vi "Write Key (Variant)__lvcfg.vi"(5 "float number format":string, 6 "write raw string? (F)":bool, 7 "section":string, 8 "error in (no error)":errorcluster, 9 "key-value":variant, 10 "key (optional)":string, 11 "Config in":T1) -> (0 "error out":errorcluster, 3 "Config out":T1)   [LabVIEW 2017, in "LabVIEW Config(Variant).lvlib"]
doc: "Writes a value associated with key in a specified section of the configuration data identified by refnum. If \"key\" input is not specified, the name of the variant object is used as the key.\n\nFor example a Boolean named \"Enable\" with a value of TRUE would correspond to the key-value pair:\n\nEnable=TRUE\n\nNote: Special characters in section and key names will be escape-coded. These include the following: \\00-\\1F (non-printable chars); \"[\", \"]\", and \"=\" (INI syntax elements); \\FE (\"þ\") and \\FF (\"ÿ\") (legacy bracket encoding); Additionally, the escape character, \"\\\", will be escaped as \"\\\\\"."
uses:
  LabVIEW Config(Variant).lvlib
  <userlib>/_NEVSTOP/Communicable State Machine(CSM)/addons/INI-Static-Variable-Support/LabVIEW-Config/Config.ctl
  <userlib>/_NEVSTOP/Communicable State Machine(CSM)/addons/INI-Static-Variable-Support/LabVIEW-Config/Write Key (Raw).vi
  <userlib>/_NEVSTOP/Communicable State Machine(CSM)/addons/INI-Static-Variable-Support/LabVIEW-Config/Write Key (String).vi
  <userlib>/_NEVSTOP/Communicable State Machine(CSM)/addons/INI-Static-Variable-Support/LabVIEW-Config/LabVIEW-Config.lvlib
  <userlib>/_NEVSTOP/Communicable State Machine(CSM)/Communicable State Machine.lvlib
panel:
  in  "Ref for recursive call":refnum<vi>
  # "Write Key (Variant).vi\n\nWrites a variant key-value to INI file.\n\nPlease visit http://www.OpenG.org to learn about the\nOpen Source LabVIEW software movement.\n\nNOTICE -- YOU MUST LEAVE THIS NOTICE IN PLACE.  PER THE TERMS OF THE LICENSE BELOW, YOU MAY SUBLICENSE THIS SOFTWARE \nIN ANY WAY THAT DOES NOT CONFLICT WITH THIS LICENSE.\n\n### BSD License (http://www.opensource.org/licenses/bsd-license.php) Begin ###\n \nCopyright (c) 2002, Jean-Pierre Drolet <drolet_jp@hotmail.com>\nCopyright (c) 2002-2006, Jim Kring <jim@jimkring.com>\n\nAll rights reserved.\n\nRedistribution and use in source and binary forms, with or without modification, are permitted provided that the following conditions are met:\n\n    * Redistributions of source code must retain the above copyright notice, this list of conditions and the following disclaimer.\n    * Redistributions in binary form must reproduce the above copyright notice, this list of conditions and the following disclaimer in the \n       documentation and/or other materials provided with the distribution.\n    * Neither the name of SciWare, James Kring, Inc., nor the names of its contributors may be used to endorse or promote products derived \n       from this software without specific prior written permission.\n\nTHIS SOFTWARE IS PROVIDED BY THE COPYRIGHT HOLDERS AND CONTRIBUTORS \"AS IS\" AND ANY EXPRESS OR IMPLIED WARRANTIES, \nINCLUDING, BUT NOT LIMITED TO, THE IMPLIED WARRANTIES OF MERCHANTABILITY AND FITNESS FOR A PARTICULAR PURPOSE ARE \nDISCLAIMED. IN NO EVENT SHALL THE COPYRIGHT OWNER OR CONTRIBUTORS BE LIABLE FOR ANY DIRECT, INDIRECT, INCIDENTAL,\n SPECIAL, EXEMPLARY, OR CONSEQUENTIAL DAMAGES (INCLUDING, BUT NOT LIMITED TO, PROCUREMENT OF SUBSTITUTE GOODS OR \nSERVICES; LOSS OF USE, DATA, OR PROFITS; OR BUSINESS INTERRUPTION) HOWEVER CAUSED AND ON ANY THEORY OF LIABILITY, \nWHETHER IN CONTRACT, STRICT LIABILITY, OR TORT (INCLUDING NEGLIGENCE OR OTHERWISE) ARISING IN ANY WAY OUT OF THE USE \nOF THIS SOFTWARE, EVEN IF ADVISED OF THE POSSIBILITY OF SUCH DAMAGE.\n\n### BSD License End ###"
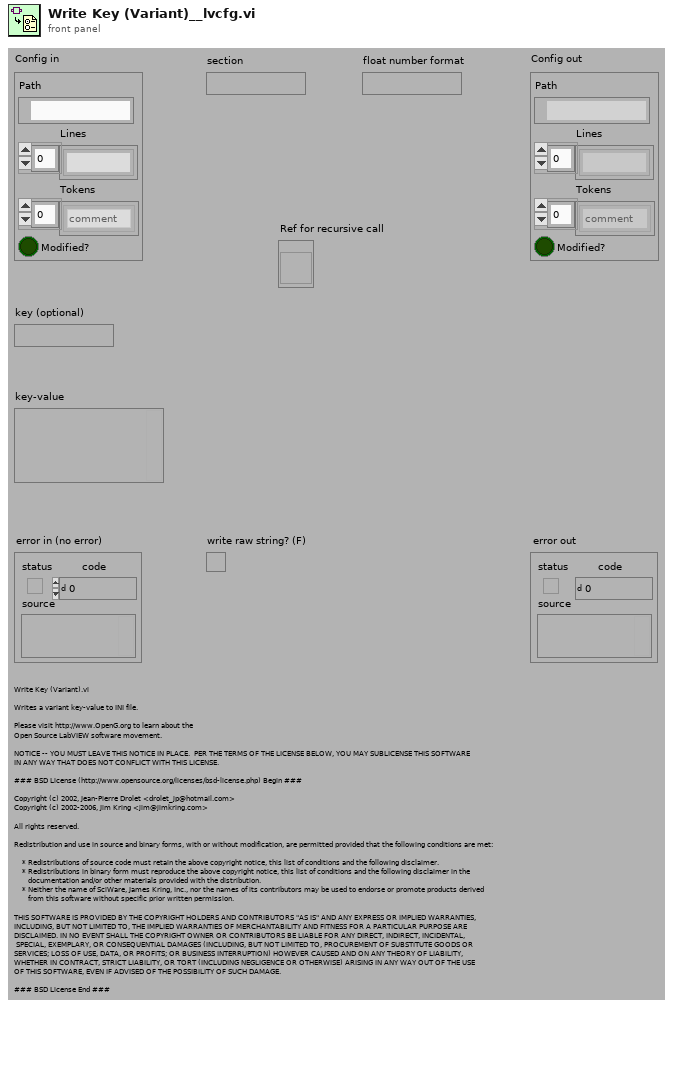
[diagram p1: front panel]
types:
  T1 = typedef "LabVIEW-Config.lvlib/Config.ctl" = cluster{"Path":path, "Lines":string[], "Tokens":enum8{"comment", "section", "key"}[], "Modified?":bool}
  T2 = typedef "Type Descriptor Enumeration__ogtk.ctl" = enum8{"<Null>", "I8", "I16", "I32", "I64", "U8", "U16", "U32", "U64", "SGL", "DBL", "EXT", "CSG", "CDB", "CXT", "0x0F", "0x10", "0x11", "0x12", "0x13", "0x14", "Enum U8", "Enum U16", "Enum U32", "Enum U64", "SGL PQ", "DBL PQ", "EXT PQ", "CSG PQ", "CDB PQ", "CXT PQ", "0x1F", "0x20", "Boolean", "0x22", "0x23", "0x24", "0x25", "0x26", "0x27", "0x28", "0x29", "0x2A", "0x2B", "0x2C", "0x2D", "0x2E", "0x2F", "String", "0x31", "Path", "Pict", "0x34", "0x35", "0x36", "DAQ", "0x38", "0x39", "0x3A", "0x3B", "0x3C", "0x3D", "0x3E", "0x3F", "Array", "0x41", "0x42", "0x43", "0x44", "0x45", "0x46", "0x47", "0x48", "0x49", "0x4A", "0x4B", "0x4C", "0x4D", "0x4E", "0x4F", "Cluster", "0x51", "0x52", "Variant", "Waveform", "0x55", "0x56", "0x57", "0x58", "0x59", "0x5A", "0x5B", "0x5C", "0x5D", "0x5E", "Fixed Point", "0x60", "0x61", "0x62", "0x63", "0x64", "0x65", "0x66", "0x67", "0x68", "0x69", "0x6A", "0x6B", "0x6C", "0x6D", "0x6E", "0x6F", "Refnum", "0x71", "0x72", "Set Collection", "Map Collection"}
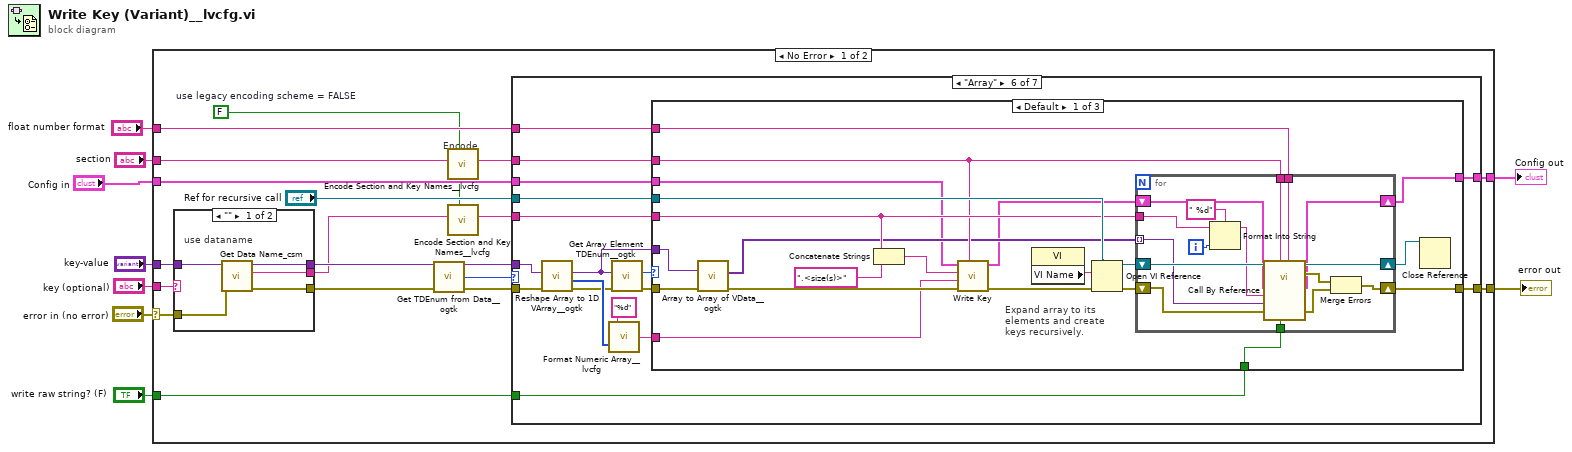
[diagram p0: block diagram]
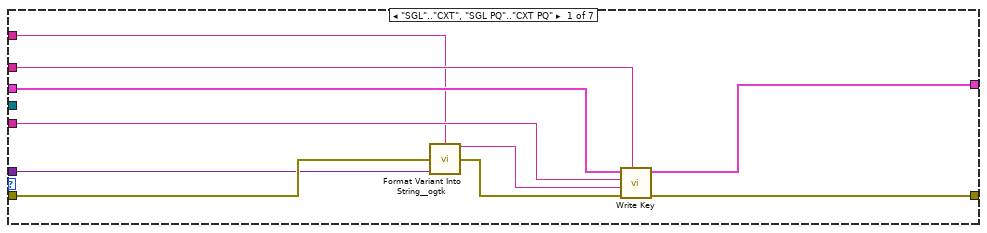
[diagram p2: hidden frame]
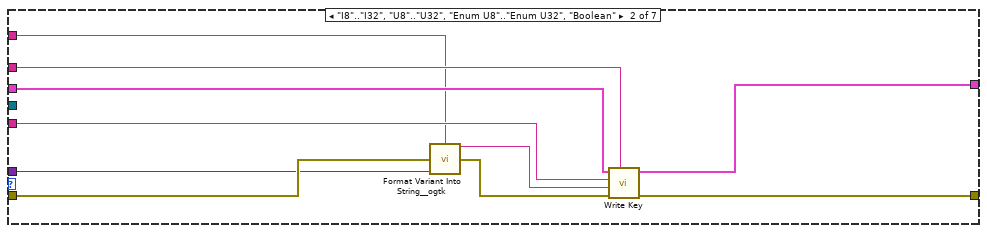
[diagram p3: hidden frame]
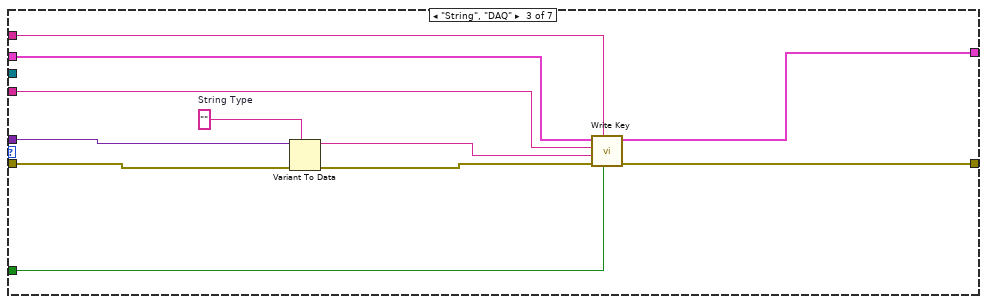
[diagram p4: hidden frame]
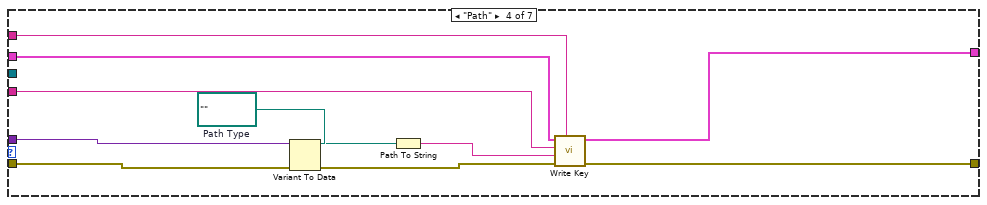
[diagram p5: hidden frame]
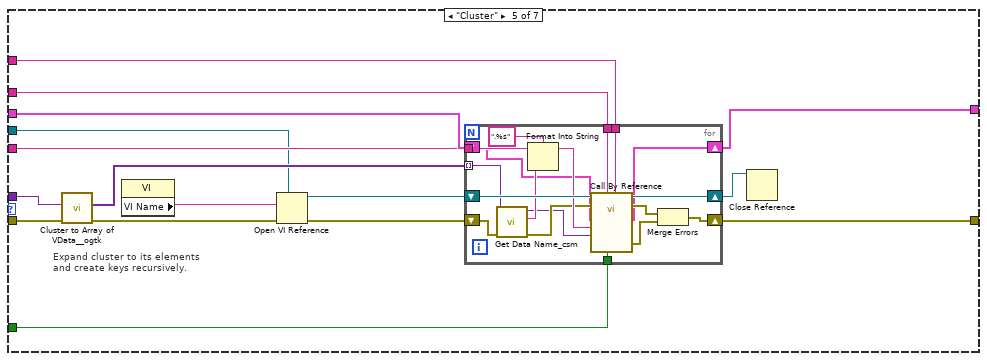
[diagram p6: hidden frame]
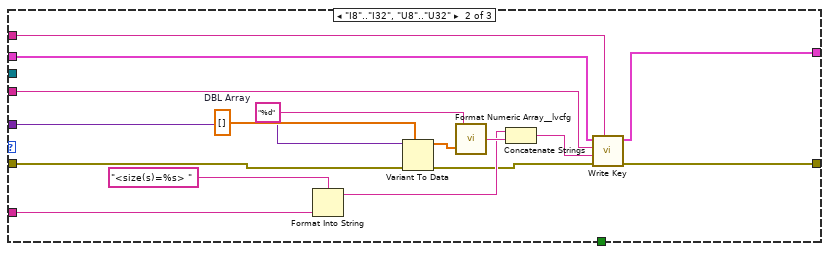
[diagram p7: hidden frame]
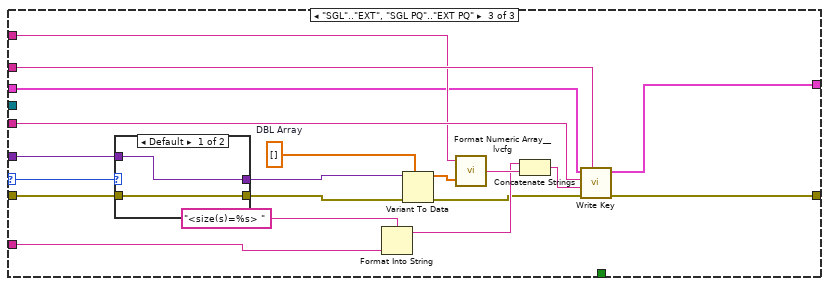
[diagram p8: hidden frame]
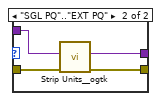
[diagram p9: hidden frame]
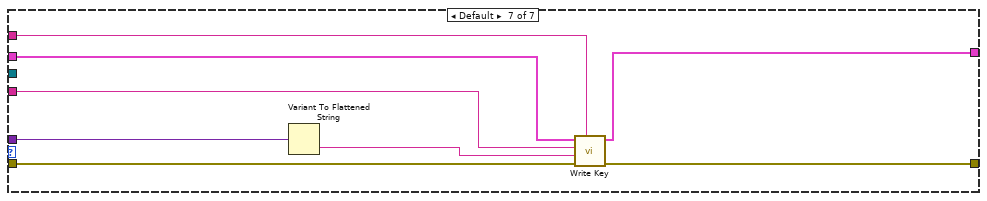
[diagram p10: hidden frame]
diagram:
  n1 = case shown="No Error" "error in (no error)" {
    selector: "error in (no error)" -> [w23 w215]
    tunnel: "Config in" -> [w26 w214]
    tunnel: [w25 w215] -> w9
    tunnel: "key-value" -> [w20 _]
    tunnel: "key (optional)" -> [w24 _]
    tunnel: "section" -> [w15 _]
    tunnel: "float number format" -> [w17 _]
    tunnel: "write raw string? (F)" -> [w16 _]
    tunnel: [w10 w214] -> w1
    frame No Error {
      w11 = FALSE  # use legacy encoding scheme = FALSE
      # "Encode"
      n2 = case shown="\"\"" w24 {
        selector: w24 -> [_ w213]
        tunnel: [w210 w213] -> w13
        tunnel: w20 -> [w207 w211]
        tunnel: w23 -> [w209 w212]
        tunnel: [w208 w212] -> w21
        tunnel: [w206 w211] -> w19
        frame "" {
          # "use dataname"
          n3 = call <userlib>:"Get Data Name_csm.vi"("error in (no error)"=w209, "Data"=w207) -> ("error out"=w208:errorcluster, "Data Name"=w210:string, "Data dup"=w206:variant)  [unwired: 7 in]
        }
        frame Default {
          # "use optional\nkey"
        }
      }
      n4 = call <userlib>:"Get TDEnum from Data__ogtk.vi"("Data"=w19) -> ("Type Descriptor Enumeration"=w22:T2)  [unwired: 4 in]
      n5 = call "Encode Section and Key Names__lvcfg.vi"("use legacy encoding scheme? (FALSE)"=w11, "string"=w15) -> ("encoded string"=w14:string)  [unwired: 9 in]
      n6 = call "Encode Section and Key Names__lvcfg.vi"("use legacy encoding scheme? (FALSE)"=w11, "string"=w13) -> ("encoded string"=w12:string)  [unwired: 9 in]
      n7 = case shown="\"Array\"" w22 {
        tunnel: w19 -> [w32 w42 w55 w67 w77 w117 w202]
        tunnel: w26 -> [w30 w39 w48 w60 w81 w111 w199]
        tunnel: [w36 w46 w53 w65 w79 w119 w205] -> w25
        tunnel: w21 -> [w33 w43 w52 w64 w76 w116 w201]
        tunnel: w12 -> [w35 w45 w51 w63 w73 w110 w204]
        tunnel: w14 -> [w34 w44 w50 w62 w80 w112 w203]
        tunnel: "Ref for recursive call" -> [_ _ _ _ w72 w118 _]
        tunnel: w17 -> [w27 w37 _ _ w71 w105 _]
        tunnel: w16 -> [_ _ w49 _ w70 w104 _]
        tunnel: [w28 w38 w47 w58 w69 w103 w198] -> w10
        frame "SGL".."CXT", "SGL PQ".."CXT PQ" {
          n8 = call <userlib>:"Format Variant Into String__ogtk.vi"("Format String"=w27, "error in (no error)"=w33, "Variant"=w32) -> ("Output String"=w29:string, "error out"=w31:errorcluster)  [unwired: 11 in]
          n9 = call-poly <userlib>:"Write Key.vi"("Section Name"=w34, "error in (no error)"=w31, "Value"=w29, "Key Name"=w35, "Config in"=w30) -> ("error out"=w36:errorcluster, "Config out"=w28:T1)  [unwired: 4 in, 1 out]
        }
        frame "I8".."I32", "U8".."U32", "Enum U8".."Enum U32", "Boolean" {
          n10 = call <userlib>:"Format Variant Into String__ogtk.vi"("Format String"=w37, "error in (no error)"=w43, "Variant"=w42) -> ("Output String"=w40:string, "error out"=w41:errorcluster)  [unwired: 11 in]
          n11 = call-poly <userlib>:"Write Key.vi"("Section Name"=w44, "error in (no error)"=w41, "Value"=w40, "Key Name"=w45, "Config in"=w39) -> ("error out"=w46:errorcluster, "Config out"=w38:T1)  [unwired: 4 in, 1 out]
        }
        frame "String", "DAQ" {
          w57 = ""  # String Type
          n12 = Variant To Data(error in=w52, type=w57, Variant=w55) -> (data=w56:string, error out=w54:errorcluster)
          n13 = call-poly <userlib>:"Write Key.vi"("Write Raw String? (F)"=w49, "Section Name"=w50, "error in (no error)"=w54, "Value"=w56, "Key Name"=w51, "Config in"=w48) -> ("error out"=w53:errorcluster, "Config out"=w47:T1)  [unwired: 3 in, 1 out]
        }
        frame "Path" {
          w68 = path ""  # Path Type
          n14 = Variant To Data(error in=w64, type=w68, Variant=w67) -> (data=w61:path, error out=w66:errorcluster)
          n15 = Path To String(path=w61) -> (string=w59:string)
          n16 = call-poly <userlib>:"Write Key.vi"("Section Name"=w62, "error in (no error)"=w66, "Value"=w59, "Key Name"=w63, "Config in"=w60) -> ("error out"=w65:errorcluster, "Config out"=w58:T1)  [unwired: 4 in, 1 out]
        }
        frame "Cluster" {
          # "Expand cluster to its elements\nand create keys recursively."
          n17 = call <userlib>:"Cluster to Array of VData__ogtk.vi"("error in (no error)"=w76, "Cluster"=w77) -> ("error out"=w74:errorcluster, "Array of VData"=w75:variant[])  [unwired: 8 in]
          n18 = property class="VI"() -> ("VI Name"=w78:string)  [unwired: 2 in, 2 out]
          n19 = Open VI Reference(type specifier VI Refnum (for type only)=w72, vi path=w78, error in (no error)=w74) -> (vi reference=w84:refnum<vi>, error out=w82:errorcluster)  [unwired: 3 in]
          n20 = for {
            shift-right: [w101] -> w83
            shift-left: w84 -> [w102]
            shift-right: [w97] -> w79
            shift-left: w82 -> [w92]
            tunnel: w75 -> [w90] mode=indexing
            tunnel: w80 -> [w100]
            tunnel: w73 -> [w96]
            tunnel: w71 -> [w88]
            tunnel: w70 -> [w86]
            shift-right: [w85] -> w69
            shift-left: w81 -> [w87]
            n21 = call <userlib>:"Get Data Name_csm.vi"("error in (no error)"=w92, "Data"=w90) -> ("error out"=w91:errorcluster, "Data Name"=w95:string, "Data dup"=w89:variant)  [unwired: 7 in]
            n22 = Format Into String(format string=".%s" ("Format String"), initial string=w96, w95) -> (resulting string=w94:string)  [unwired: 1 in, 1 out]
            n23 = call-by-ref "?"(reference=w102, error in=w91, "float number format"=w88, "write raw string? (F)"=w86, "section"=w100, "key-value"=w89, "key (optional)"=w94, "Config in"=w87) -> (reference out=w101:refnum<vi>, error out=w98:errorcluster, "error out"=w99:errorcluster, "Config out"=w85:T1)  [unwired: 4 in]
            n24 = Merge Errors(w98, w99) -> (w97:errorcluster)
          }
          n25 = Close Reference(reference=w83) -> ()  [unwired: 1 in, 1 out]
        }
        frame "Array" {
          n26 = call <userlib>:"Reshape Array to 1D VArray__ogtk.vi"("error in (no error)"=w116, "MultiD Array"=w117) -> ("error out"=w106:errorcluster, "Size(s)"=w114:u32[], "1D VArray"=w107:variant)  [unwired: 7 in]
          n27 = call "Format Numeric Array__lvcfg.vi"("Array"=w114, "format string"="%d") -> ("Formatted on a line"=w108:string)
          n28 = call <userlib>:"Get Array Element TDEnum__ogtk.vi"("error in (no error)"=w106, "Array"=w107) -> ("error out"=w109:errorcluster, "Element Type"=w113:T2)  [unwired: 8 in]
          n29 = case shown="Default" w113 {
            selector: w113 -> [_ _ w181]
            tunnel: w111 -> [w122 w158 w175]
            tunnel: w112 -> [w131 w163 w184]
            tunnel: [w137 w161 w182] -> w119
            tunnel: w110 -> [w134 w162 w183]
            tunnel: w118 -> [w135 _ _]
            tunnel: w109 -> [w129 w164 w180]
            tunnel: w108 -> [w123 w165 w185]
            tunnel: w107 -> [w127 w160 w178]
            tunnel: w105 -> [w125 _ w176]
            tunnel: w104 -> [w124 _ _]
            tunnel: [w120 w157 w173] -> w103
            frame Default {
              # "Expand array to its\nelements and create\nkeys recursively."
              n30 = call <userlib>:"Array to Array of VData__ogtk.vi"("error in (no error)"=w129, "MultiD Array"=w127) -> ("error out"=w128:errorcluster, "1D Array of Variants"=w126:variant[])  [unwired: 8 in]
              n31 = Concatenate Strings(w134, ".<size(s)>" ("Substring")) -> (w130:string)
              n32 = call-poly <userlib>:"Write Key.vi"("Section Name"=w131, "error in (no error)"=w128, "Value"=w123, "Key Name"=w130, "Config in"=w122) -> ("error out"=w133:errorcluster, "Config out"=w121:T1)  [unwired: 4 in, 1 out]
              n33 = property class="VI"() -> ("VI Name"=w136:string)  [unwired: 2 in, 2 out]
              n34 = Open VI Reference(type specifier VI Refnum (for type only)=w135, vi path=w136, error in (no error)=w133) -> (vi reference=w140:refnum<vi>, error out=w138:errorcluster)  [unwired: 3 in]
              n35 = for {
                shift-right: [w155] -> w139
                shift-left: w140 -> [w156]
                shift-right: [w151] -> w137
                shift-left: w138 -> [w146]
                tunnel: w126 -> [w147] mode=indexing
                tunnel: w131 -> [w154]
                tunnel: w134 -> [w150]
                tunnel: w125 -> [w144]
                tunnel: w124 -> [w142]
                shift-right: [w141] -> w120
                shift-left: w121 -> [w143]
                i -> [w145]
                n36 = Format Into String(format string=" %d" ("Format String"), initial string=w150, w145) -> (resulting string=w149:string)  [unwired: 1 in, 1 out]
                n37 = call-by-ref "?"(reference=w156, "float number format"=w144, "write raw string? (F)"=w142, "section"=w154, "error in (no error)"=w146, "key-value"=w147, "key (optional)"=w149, "Config in"=w143) -> (reference out=w155:refnum<vi>, error out=w152:errorcluster, "error out"=w153:errorcluster, "Config out"=w141:T1)  [unwired: 4 in]
                n38 = Merge Errors(w152, w153) -> (w151:errorcluster)
              }
              n39 = Close Reference(reference=w139) -> ()  [unwired: 1 in, 1 out]
            }
            frame "I8".."I32", "U8".."U32" {
              w172 = dbl[] []  # DBL Array
              n40 = Format Into String(format string="<size(s)=%s> " ("Format String"), w165) -> (resulting string=w167:string)  [unwired: 2 in, 1 out]
              n41 = Variant To Data(error in=w164, type=w172, Variant=w160) -> (data=w171:dbl[], error out=w166:errorcluster)
              n42 = call "Format Numeric Array__lvcfg.vi"("Array"=w171, "format string"="%d") -> ("Formatted on a line"=w170:string)
              n43 = Concatenate Strings(w167, w170) -> (w159:string)
              n44 = call-poly <userlib>:"Write Key.vi"("Section Name"=w163, "error in (no error)"=w166, "Value"=w159, "Key Name"=w162, "Config in"=w158) -> ("error out"=w161:errorcluster, "Config out"=w157:T1)  [unwired: 4 in, 1 out]
            }
            frame "SGL".."EXT", "SGL PQ".."EXT PQ" {
              w191 = dbl[] []  # DBL Array
              n45 = case shown="Default" w181 {
                tunnel: w180 -> [w193 w197]
                tunnel: [w193 w196] -> w179
                tunnel: w178 -> [w192 w195]
                tunnel: [w192 w194] -> w177
                frame Default {
                }
                frame "SGL PQ".."EXT PQ" {
                  n46 = call <userlib>:"Strip Units__ogtk.vi"("error in (no error)"=w197, "Number or 1D array with units"=w195) -> ("error out"=w196:errorcluster, "Pure Number(s) (base units)"=w194:variant)  [unwired: 8 in]
                }
              }
              n47 = Format Into String(format string="<size(s)=%s> " ("Format String"), w185) -> (resulting string=w187:string)  [unwired: 2 in, 1 out]
              n48 = Variant To Data(error in=w179, type=w191, Variant=w177) -> (data=w190:dbl[], error out=w186:errorcluster)
              n49 = call "Format Numeric Array__lvcfg.vi"("Array"=w190, "format string"=w176) -> ("Formatted on a line"=w189:string)
              n50 = Concatenate Strings(w187, w189) -> (w174:string)
              n51 = call-poly <userlib>:"Write Key.vi"("Section Name"=w184, "error in (no error)"=w186, "Value"=w174, "Key Name"=w183, "Config in"=w175) -> ("error out"=w182:errorcluster, "Config out"=w173:T1)  [unwired: 4 in, 1 out]
            }
          }
        }
        frame Default {
          n52 = Variant To Flattened String(Variant=w202) -> (data string=w200:string)  [unwired: 1 out]
          n53 = call-poly <userlib>:"Write Key.vi"("Section Name"=w203, "error in (no error)"=w201, "Content"=w200, "Key Name"=w204, "Config in"=w199) -> ("error out"=w205:errorcluster, "Config out"=w198:T1)  [unwired: 4 in, 1 out]
        }
      }
    }
    frame Error {
    }
  }
  "error out" <- w9
  "Config out" <- w1
